vi "HFRR ADV v13.vi"() -> ()   [LabVIEW 2025] (continued)
              }
              frame True {
                n1529 = Delete From Array(array=w2011, length=w2010, index=0) -> (array with subset deleted=w2012:dbl[])  [unwired: 1 out]
                "Numeric" <- w2010
              }
            }
            "FF1" <- w1997
            "PID Ref" <- TRUE ("PID Ref")
          }
          frame #2 {
          }
          frame #3 {
            # "CONVERT TO N"
            # "DATA PROCESSING"
            # "115 mV/N"
            n1530 = local read "RH Numeric:"() -> (w2018:dbl)
            n1531 = local read "HUMIDITY:"() -> (w2019:dbl)
            n1532 = local read "temp buf"() -> (w2080:dbl[])
            n1533 = local read "Air temp"() -> (w2078:dbl[])
            n1534 = local read "ecr buf"() -> (w2040:dbl[])
            n1535 = local read "Fric Val"() -> (w2083:dbl[])
            n1536 = case shown="True" "Reset Button" {
              frame False {
              }
              frame True {
                n1537 = local write "Reset Button"(FALSE) -> ()
                n1538 = local write "Captured Values"(dbl[][] [] ("Captured Values")) -> ()
                n1539 = local write "Best Fit"(dbl[] [] ("Best Fit")) -> ()
              }
            }
            n1540 = local read "TEMPERATURE :"() -> (w2061:dbl)
            n1541 = call-poly <vilib>:"Mean.vi"("X"=w2040) -> ("mean"=w2037:dbl)  [unwired: 1 out]
            n1542 = call-poly <vilib>:"Mean.vi"("X"=w2078) -> ("mean"=w2047:dbl)  [unwired: 1 out]
            "Raw air temp" <- w2047
            n1543 = call-poly <vilib>:"Mean.vi"("X"=w2080) -> ("mean"=w2049:dbl)  [unwired: 1 out]
            "Raw specimen temp" <- w2049
            n1544 = local read "TEMP INTERCEPT:"() -> (w2054:dbl)
            n1545 = Multiply(x=w2018, y=w2019) -> (x*y=→"Humidity ( %RH )" →"Hum" →"Hum 2":dbl)
            n1546 = Multiply(x=w2083, y=1.0) -> (x*y=w2084:dbl[])
            n1547 = local read "FRIC. FORCE :"() -> (w2077:dbl)
            n1548 = Multiply(x=w2049, y=w2061) -> (x*y=w2043:dbl)
            n1549 = local read "AIR TEMPERATURE :"() -> (w2062:dbl)
            n1550 = local read "RUN"() -> (w2074:bool)
            n1551 = Add(x=w2047, y="Offset Air Temp") -> (x+y=w2042:dbl)
            n1552 = local read "AIR TEMP INTERCEPT:"() -> (w2058:dbl)
            n1553 = case shown="\"0\", Default" "Calibrating" {
              tunnel: w2049 -> [w2103 _]
              tunnel: [w2103 w2104] -> w2048
              tunnel: w2047 -> [_ w2104]
              frame "0", Default {
              }
              frame "1" {
              }
            }
            n1554 = Multiply(x=w2037, y="ECR_Gain") -> (x*y=w2036:dbl)
            n1555 = Add(x=w2043, y=w2054) -> (x+y=w2059:dbl)
            n1556 = Multiply(x=w2077, y=79.77669138) -> (x*y=w2075:dbl)
            n1557 = Select(t=0.01 ("FF fil1"), s=w2074, f=0.1 ("FF fil1")) -> (s? t:f=w2070:dbl)
            n1558 = local read "ecr"() -> (w2031:dbl)
            n1559 = Multiply(x=w2042, y=w2062) -> (x*y=w2044:dbl)
            n1560 = Multiply(x=w2084, y=w2075) -> (x*y=w2081:dbl[])
            n1561 = Multiply(x=w2036, y=0.2) -> (x*y=w2029:dbl)
            n1562 = Multiply(x=0.8, y=w2031) -> (x*y=w2030:dbl)
            n1563 = call <vilib>:"Mean PtByPt.vi"("x"=w2059, "sample length"=10) -> ("mean"=w2020:dbl)  [unwired: 2 in, 1 out]
            "TEMP 2" <- w2020
            "TEMP 3" <- w2020
            n1564 = local read "AIR TEMP"() -> (w2067:dbl)
            n1565 = Add(x=w2044, y=w2058) -> (x+y=w2060:dbl)
            n1566 = call-poly <vilib>:"Mean.vi"("X"=w2081) -> ("mean"=w2082:dbl)  [unwired: 1 out]
            n1567 = Add(x=w2029, y=w2030) -> (x+y=w2028:dbl)
            n1568 = Subtract(x=1.0 ("y"), y=w2070) -> (x-y=w2068:dbl)
            n1569 = local write "TEMP"(w2020) -> ()
            n1570 = Multiply(x=w2068, y=w2067) -> (x*y=w2066:dbl)
            n1571 = Multiply(x=w2060, y=w2070) -> (x*y=w2071:dbl)
            n1572 = Not A Number/Path/Refnum?(number/path/refnum=w2028) -> (NaN/Path/Refnum?=w2038:bool)
            n1573 = Subtract(x=w2081, y=w2082) -> (x-y=w2053:dbl[])
            n1574 = local read "FRICVALZ"() -> (w2091:dbl)
            n1575 = case shown="True" "Camera Button" {
              tunnel: w2048 -> [_ w2110]
              tunnel: "Standard Temp. ( °c )" -> [_ w2109]
              frame False {
              }
              frame True {
                n1576 = Build Array(w2109, w2110) -> (w2108:dbl[])
                n1577 = local write "Camera Button"(FALSE ("Boolean 4")) -> ()
                n1578 = local read "Captured Values"() -> (w2107:dbl[][])
                n1579 = Build Array (concatenate)(w2107, w2108) -> (w2105:dbl[][])
                n1580 = local write "Captured Values"(w2105) -> ()
              }
            }
            n1581 = Compound Arithmetic op=OR("FRICVALZ 4", "FRICVALZ 3", "FRICVALZ 2") -> (w2022:bool)
            n1582 = Add(x=w2071, y=w2066) -> (x+y=w2064:dbl)
            n1583 = Absolute Value(x=w2053) -> (abs(x)=w2086:dbl[])
            n1584 = call-poly <vilib>:"RMS.vi"("X"=w2053) -> ("rms value"=w2052:dbl)  [unwired: 1 out]
            n1585 = Select(t=0.0, s=w2038, f=w2028) -> (s? t:f=w2035:dbl)
            n1586 = call-poly <vilib>:"Mean.vi"("X"=w2086) -> ()  [unwired: 2 out]
            n1587 = local read "FF 2"() -> (w2093:dbl)
            n1588 = case shown="True" w2022 {
              tunnel: w2052 -> [_ w2115]
              frame False {
              }
              frame True {
                w2114 = FALSE ("FRICVALZ")
                n1589 = local write "FRICVALZ 3"(w2114) -> ()
                n1590 = local write "FRICVALZ 2"(w2114) -> ()
                n1591 = local write "FRICVALZ 4"(w2114) -> ()
                "FRICVALZ" <- w2115
              }
            }
            n1592 = Subtract(x=w2052, y=w2091) -> (x-y=w2085:dbl)
            n1593 = Not A Number/Path/Refnum?(number/path/refnum=w2064) -> (NaN/Path/Refnum?=w2065:bool)
            n1594 = In Range and Coerce(upper limit=100.0, x=w2035, lower limit=0.0) -> ()  [unwired: 2 out]
            n1595 = Select(t=0.0, s=w2065, f=w2064) -> (s? t:f=w2025:dbl)
            "AIR TEMP" <- w2025
            n1596 = Multiply(x=w2085, y=0.1 ("FF fil1")) -> (x*y=w2097:dbl)
            n1597 = Multiply(x=0.9 ("FF fil2"), y=w2093) -> (x*y=w2096:dbl)
            n1598 = disable-structure shown="Disabled" {
              frame Disabled {
                n1599 = local read "NORMAL LOAD"() -> ()  [unwired: 1 out]
              }
              frame Enabled {
              }
            }
            n1600 = call "Elapsed Time11"("Time Target (s)"=1.0) -> ("Time has Elapsed"=w2027:bool)  [unwired: 11 in, 7 out]
            n1601 = Add(x=w2097, y=w2096) -> (x+y=w2015:dbl)
            "FF 2" <- w2015
            "FF 4" <- w2015
            n1602 = case shown="True" w2027 {
              tunnel: w2025 -> [_ w2099]
              frame False {
              }
              frame True {
                "AirT" <- w2099
              }
            }
            n1603 = local read "TEMP"() -> (w2090:dbl)
            n1604 = local write "FF 3"(w2015) -> ()
            n1605 = Not A Number/Path/Refnum?(number/path/refnum=w2015) -> (NaN/Path/Refnum?=w2088:bool)
            n1606 = Divide(x=w2015, y=1.96) -> (x/y=w2055:dbl)
            n1607 = Not A Number/Path/Refnum?(number/path/refnum=w2090) -> (NaN/Path/Refnum?=w2089:bool)
            n1608 = Compound Arithmetic op=OR(w2089, w2088) -> (w2087:bool)
            n1609 = Not A Number/Path/Refnum?(number/path/refnum=w2055) -> (NaN/Path/Refnum?=w2056:bool)
            n1610 = case shown="True" w2087 {
              frame False {
              }
              frame True {
                n1611 = local write "TEMP"(0.0 ("TEMP")) -> ()
                n1612 = local write "FF 2"(0.0 ("FF 2")) -> ()
                n1613 = local write "reinit"(TRUE ("reinit")) -> ()
              }
            }
            n1614 = Select(t=0.0, s=w2056, f=w2055) -> (s? t:f=w2016:dbl)
            "COF 2" <- w2016
            n1615 = local write "COF 3"(w2016) -> ()
          }
          frame #4 {
            n1616 = flat-sequence {
              frame #0 {
                n1617 = Wait (ms)(milliseconds to wait=u32 100) -> ()  [unwired: 1 out]
              }
              frame #1 {
                n1618 = local write "Lift"(FALSE ("Lift")) -> ()
              }
            }
            n1619 = case shown="True" "Calculate Button" {
              frame False {
              }
              frame True {
                n1620 = local write "Calculate Button"(FALSE ("Boolean 6")) -> ()
                n1621 = local read "Captured Values"() -> (w2126:dbl[][])
                n1622 = Index Array(array=w2126, index (col) #1=0 ("disabled index (col)"), index (col) #2=1 ("index (col)")) -> (element #1=w2124:dbl[], element #2=w2122:dbl[])  [unwired: 2 in]
                n1623 = call <vilib>:"Linear Fit.vi"("Y"=w2124, "X"=w2122) -> ("Best Linear Fit"=→"Best Fit":dbl[], "slope"=w2118:dbl, "intercept"=w2117:dbl)  [unwired: 9 in, 2 out]
                "Slope" <- w2118
                "Intercept" <- w2117
                n1624 = local read "Calibrating"() -> (w2119:string)
                n1625 = case shown="\"1\"" w2119 {
                  tunnel: w2118 -> [w2128 w2130]
                  tunnel: w2117 -> [w2127 w2129]
                  frame "0", Default {
                    n1626 = local write "TEMPERATURE :"(w2128) -> ()
                    n1627 = local write "TEMP INTERCEPT:"(w2127) -> ()
                  }
                  frame "1" {
                    n1628 = local write "AIR TEMPERATURE :"(w2130) -> ()
                    n1629 = local write "AIR TEMP INTERCEPT:"(w2129) -> ()
                  }
                }
              }
            }
          }
        }
      }
    }
    n1630 = Wait (ms)(milliseconds to wait=u32 50) -> ()  [unwired: 1 out]
    n1631 = local read "Quit"() -> (w1920:bool)
    "Rate" <- 2500.0 ("No of Samples")
    "Humid Last buf" <- dbl[] [0.0, 0.0, 0.0, 0.0] ("Humid Last buf")
  }
  n1632 = while {
    tunnel: w60 -> [_]
    tunnel: [w2160] -> _
    tunnel: [w2135] -> w57
    i -> [w2160]
    stop <- w2135 stop-if-true
    # "C:\\LAB-IQ-NXT\\Scar View.exe"
    n1633 = local read "OK Button 16"() -> (w2149:bool)
    n1634 = local read "Re-Initialise"() -> (w2145:bool)
    n1635 = local read "Main Tab"() -> (w2141:T2)
    n1636 = local read "service 3"() -> (w2142:bool)
    n1637 = local read "OPEN 6"() -> (w2144:bool)
    n1638 = local read "EDIT 2"() -> (w2147:bool)
    n1639 = flat-sequence {
      frame #0 {
        n1640 = local read "SAVE 2"() -> (w2763:bool)
        n1641 = stacked-sequence {
          frame #0 {
            n1642 = local read "EDIT"() -> (w2817:bool)
            n1643 = case shown="True" w2817 {
              tunnel: [u8 2 ("Disabled") u8 0 ("Disabled")] -> _
              frame False {
                w2819 = FALSE
                n1644 = local write "Password"("") -> ()
                n1645 = property on="SrvM CP" class="Bool (strict)"("Visible"=w2819) -> ()  [unwired: 2 in, 2 out]
                n1646 = property on="message" class="Str"("Visible"=w2819) -> ()  [unwired: 2 in, 2 out]
                n1647 = local write "x = y?"(w2819) -> ()
                n1648 = property on="Password" class="Str"("Visible"=w2819) -> ()  [unwired: 2 in, 2 out]
                n1649 = property on="ENTER THE NEW PASSWORD" class="Str"("Visible"=w2819) -> ()  [unwired: 2 in, 2 out]
                n1650 = property on="ENTER CURRENT PASSWORD" class="Str"("Visible"=w2819) -> ()  [unwired: 2 in, 2 out]
                n1651 = local write "SrvM CP"(w2819) -> ()
              }
              frame True {
                w2822 = TRUE
                n1652 = property on="SrvM CP" class="Bool (strict)"("Visible"=w2822) -> ()  [unwired: 2 in, 2 out]
                n1653 = property on="Password" class="Str"("Visible"=w2822) -> ()  [unwired: 2 in, 2 out]
              }
            }
            "dipl pwd" <- "@143$\n" ("dipl pwd")
          }
          frame #1 {
            # "Gain password"
            n1654 = String To Byte Array(string="ENTER CURRENT PASSWORD") -> (unsigned byte array=w2827:u8[])
            n1655 = Search 1D Array(1D array=w2827, element=u8 10) -> (index of element=w2830:i32)  [unwired: 1 in]
            n1656 = Index Array(array=w2827, index=w2830) -> (element=w2826:u8)
            n1657 = Equal?(x=w2826, y=10) -> (x = y?=w2824:bool)
            n1658 = case shown="True" w2824 {
              frame False {
                n1659 = property on="ENTER THE NEW PASSWORD" class="Str"("Visible"=FALSE) -> ()  [unwired: 2 in, 2 out]
              }
              frame True {
                # "password"
                # "change password logic"
                n1660 = local read "ENTER CURRENT PASSWORD"() -> (w2843:string)
                n1661 = local read "dipl pwd"() -> (w2837:string)
                n1662 = String To Byte Array(string=w2843) -> (unsigned byte array=w2845:u8[])
                n1663 = String To Byte Array(string=w2837) -> (unsigned byte array=w2838:u8[])
                n1664 = Array Size(array=w2845) -> (size(s)=w2842:i32)
                n1665 = Array Size(array=w2838) -> (size(s)=w2840:i32)
                n1666 = for {
                  N: w2842 -> [_]
                  tunnel: w2845 -> [w2869]
                  tunnel: [w2867] -> w2846 mode=indexing
                  tunnel: w2842 -> [w2861]
                  i -> [w2862]
                  n1667 = Decrement(x=w2861) -> (x-1=w2859:i32)
                  n1668 = Equal?(x=w2862, y=w2859) -> (x = y?=w2860:bool)
                  n1669 = Index Array(array=w2869, index=w2862) -> (element=w2863:u8)
                  n1670 = Number To Decimal String(number=w2863) -> (decimal integer string=w2868:string)  [unwired: 1 in]
                  n1671 = Select(t="", s=w2860, f="\r") -> (s? t:f=w2865:string)
                  n1672 = Concatenate Strings(w2868, w2865) -> (w2867:string)
                }
                n1673 = for {
                  N: w2840 -> [_]
                  tunnel: w2838 -> [w2857]
                  tunnel: [w2855] -> w2839 mode=indexing
                  tunnel: w2840 -> [w2852]
                  i -> [w2853]
                  n1674 = Decrement(x=w2852) -> (x-1=w2851:i32)
                  n1675 = Equal?(x=w2853, y=w2851) -> (x = y?=w2850:bool)
                  n1676 = Index Array(array=w2857, index=w2853) -> (element=w2856:u8)
                  n1677 = Number To Decimal String(number=w2856) -> (decimal integer string=w2854:string)  [unwired: 1 in]
                  n1678 = Select(t="", s=w2850, f="\r") -> (s? t:f=w2847:string)
                  n1679 = Concatenate Strings(w2854, w2847) -> (w2855:string)
                }
                n1680 = local read "string"() -> (w2844:string)
                n1681 = Concatenate Strings(w2839) -> (w2833:string)
                n1682 = Concatenate Strings(w2844) -> (w2841:string)
                n1683 = Concatenate Strings(w2846) -> (w2834:string)
                n1684 = Equal?(x=w2834, y=w2841) -> (x = y?=w2836:bool)
                n1685 = Equal?(x=w2834, y=w2833) -> (x = y?=w2832:bool)
                n1686 = Or(x=w2836, y=w2832) -> (x .or. y?=w2835:bool)
                n1687 = case shown="True" w2835 {
                  frame False {
                  }
                  frame True {
                    n1688 = property on="ENTER THE NEW PASSWORD" class="Str"("Visible"=TRUE) -> ()  [unwired: 2 in, 2 out]
                  }
                }
              }
            }
          }
          frame #2 {
            n1689 = String To Byte Array(string="ENTER THE NEW PASSWORD") -> (unsigned byte array=w2872:u8[])
            n1690 = Search 1D Array(1D array=w2872, element=u8 10) -> (index of element=w2876:i32)  [unwired: 1 in]
            n1691 = Index Array(array=w2872, index=w2876) -> (element=w2874:u8)
            n1692 = Equal?(x=w2874, y=10) -> (x = y?=w2871:bool)
            n1693 = case shown="False" w2871 {
              frame False {
              }
              frame True {
                n1694 = local write "EDIT"(FALSE) -> ()
                n1695 = local write "SrvM CP"(FALSE) -> ()
                n1696 = local read "ENTER THE NEW PASSWORD"() -> (w2879:string)
                n1697 = String To Byte Array(string=w2879) -> (unsigned byte array=w2884:u8[])
                n1698 = Array Size(array=w2884) -> (size(s)=w2881:i32)
                n1699 = for {
                  N: w2881 -> [_]
                  tunnel: w2884 -> [w2897]
                  tunnel: [w2894] -> w2886 mode=indexing
                  tunnel: w2881 -> [w2889]
                  i -> [w2887]
                  n1700 = Decrement(x=w2889) -> (x-1=w2890:i32)
                  n1701 = Equal?(x=w2887, y=w2890) -> (x = y?=w2891:bool)
                  n1702 = Index Array(array=w2897, index=w2887) -> (element=w2896:u8)
                  n1703 = Number To Decimal String(number=w2896) -> (decimal integer string=w2895:string)  [unwired: 1 in]
                  n1704 = Select(t="", s=w2891, f="\r") -> (s? t:f=w2888:string)
                  n1705 = Concatenate Strings(w2895, w2888) -> (w2894:string)
                }
                n1706 = local read "file path"() -> (w2878:path)
                n1707 = Concatenate Strings(w2886) -> (w2880:string)
                n1708 = Delete(path (use dialog)=w2878) -> (deleted path=w2882:path)  [unwired: 4 in, 2 out]
                n1709 = call <vilib>:"Write Characters To File.vi"("append to file? (new file:F)"=FALSE, "character string"=w2880, "file path (dialog if empty)"=w2882) -> ()  [unwired: 2 in, 1 out]
              }
            }
          }
          frame #3 {
            n1710 = case shown="True" "SrvM CP" {
              frame False {
                w2900 = ""
                n1711 = local write "ENTER CURRENT PASSWORD"(w2900) -> ()
                n1712 = local write "ENTER THE NEW PASSWORD"(w2900) -> ()
                n1713 = property on="ENTER CURRENT PASSWORD" class="Str"("Visible"=FALSE) -> ()  [unwired: 2 in, 2 out]
              }
              frame True {
                n1714 = property on="ENTER THE NEW PASSWORD" class="Str"() -> ("Visible"=w2901:bool)  [unwired: 2 in, 2 out]
                n1715 = Not(x=w2901) -> (.not. x?=w2902:bool)
                n1716 = property on="ENTER CURRENT PASSWORD" class="Str"("Visible"=w2902) -> ()  [unwired: 2 in, 2 out]
              }
            }
          }
          frame #4 {
            n1717 = String To Byte Array(string="Password") -> (unsigned byte array=w2909:u8[])
            n1718 = Search 1D Array(1D array=w2909, element=u8 10) -> (index of element=w2907:i32)  [unwired: 1 in]
            n1719 = Index Array(array=w2909, index=w2907) -> (element=w2908:u8)
            n1720 = Equal?(x=w2908, y=10) -> (x = y?=w2904:bool)
            n1721 = case shown="True" w2904 {
              frame False {
              }
              frame True {
                # "password"
                # "password"
                n1722 = local read "Password"() -> (w2922:string)
                n1723 = String To Byte Array(string=w2922) -> (unsigned byte array=w2925:u8[])
                n1724 = String To Byte Array(string="@143$\n") -> (unsigned byte array=w2911:u8[])
                n1725 = Array Size(array=w2925) -> (size(s)=w2920:i32)
                n1726 = Array Size(array=w2911) -> (size(s)=w2916:i32)
                n1727 = for {
                  N: w2920 -> [_]
                  tunnel: w2925 -> [w2959]
                  tunnel: [w2957] -> w2926 mode=indexing
                  tunnel: w2920 -> [w2954]
                  i -> [w2955]
                  n1728 = Decrement(x=w2954) -> (x-1=w2953:i32)
                  n1729 = Index Array(array=w2959, index=w2955) -> (element=w2958:u8)
                  n1730 = Equal?(x=w2955, y=w2953) -> (x = y?=w2952:bool)
                  n1731 = Number To Decimal String(number=w2958) -> (decimal integer string=w2956:string)  [unwired: 1 in]
                  n1732 = Select(t="", s=w2952, f="\r") -> (s? t:f=w2949:string)
                  n1733 = Concatenate Strings(w2956, w2949) -> (w2957:string)
                }
                n1734 = for {
                  N: w2916 -> [_]
                  tunnel: w2911 -> [w2970]
                  tunnel: [w2968] -> w2914 mode=indexing
                  tunnel: w2916 -> [w2965]
                  i -> [w2966]
                  n1735 = Decrement(x=w2965) -> (x-1=w2964:i32)
                  n1736 = Index Array(array=w2970, index=w2966) -> (element=w2969:u8)
                  n1737 = Equal?(x=w2966, y=w2964) -> (x = y?=w2963:bool)
                  n1738 = Number To Decimal String(number=w2969) -> (decimal integer string=w2967:string)  [unwired: 1 in]
                  n1739 = Select(t="", s=w2963, f="\r") -> (s? t:f=w2960:string)
                  n1740 = Concatenate Strings(w2967, w2960) -> (w2968:string)
                }
                n1741 = local read "file path"() -> (w2910:path)
                n1742 = call <vilib>:"Read Characters From File.vi"("file path (dialog if empty)"=w2910) -> ("character string"=w2924:string)  [unwired: 5 in, 3 out]
                "string" <- w2924
                n1743 = flat-sequence {
                  tunnel: [w2927] -> w2921
                  frame #0 {
                    w2927 = ""
                    n1744 = local write "Password"(w2927) -> ()
                  }
                }
                n1745 = Concatenate Strings(w2914) -> (w2915:string)
                n1746 = Concatenate Strings(w2924) -> (w2923:string)
                n1747 = Concatenate Strings(w2926) -> (w2918:string)
                n1748 = Equal?(x=w2918, y=w2923) -> (x = y?=w2913:bool)
                n1749 = Equal?(x=w2918, y=w2915) -> (x = y?=w2919:bool)
                n1750 = Or(x=w2913, y=w2919) -> (x .or. y?=w2912:bool)
                "x = y?" <- w2912
                n1751 = case shown="True" w2912 {
                  selector: w2912 -> [w2929 _]
                  tunnel: w2921 -> [_ _]
                  frame False {
                    n1752 = And(x=w2929, y=TRUE ("Visible")) -> (x .and. y?=w2930:bool)
                    n1753 = property on="message" class="Str"("Visible"=w2930) -> ()  [unwired: 2 in, 2 out]
                  }
                  frame True {
                    n1754 = control-ref of="This VI"() -> (w2941:refnum<vi>)
                    n1755 = property class="VI"(reference=w2941) -> (reference out=w2932:refnum<vi>, error out=w2936:errorcluster, "Panel"=w2940:refnum<vi>)  [unwired: 1 in]
                    n1756 = property on="message" class="Str"("Visible"=FALSE) -> ()  [unwired: 2 in, 2 out]
                    n1757 = property class="Pnl"(reference=w2940, error in=w2936) -> (reference out=w2934:refnum<vi>, error out=w2937:errorcluster, "Panes[]"=w2939:refnum<vi>[])
                    n1758 = for {
                      tunnel: w2939 -> [w2948] mode=indexing
                      tunnel: T18."Always On" ("Horizontal Scrollbar Visibility") -> [w2947]
                      tunnel: w2937 -> [w2944]
                      tunnel: [w2943] -> w2935
                      n1759 = property class="Pane"(reference=w2948, error in=w2944, "HorizScrollbarVisibility"=w2947) -> (reference out=w2945:refnum<vi>, error out=w2946:errorcluster)
                      n1760 = Close Reference(reference=w2945, error in (no error)=w2946) -> (error out=w2943:errorcluster)
                    }
                    n1761 = Close Reference(reference=w2934, error in (no error)=w2935) -> (error out=w2933:errorcluster)
                    n1762 = Close Reference(reference=w2932, error in (no error)=w2933) -> (error out=→"error out 6":errorcluster)
                  }
                }
              }
            }
          }
        }
        n1763 = local read "x = y?"() -> (w2769:bool)
        n1764 = local read "HUMIDITY: 2"() -> (w2771:dbl)
        n1765 = local read "HUMIDITY:"() -> (w2770:dbl)
        n1766 = property on="Port 2 Error" class="Clust (strict)"("Visible"="EDIT") -> ()  [unwired: 2 in, 2 out]
        n1767 = property on="Port 1 Error" class="Clust (strict)"("Visible"="EDIT") -> ()  [unwired: 2 in, 2 out]
        n1768 = case shown="True" "SrvM CP 2" {
          frame False {
          }
          frame True {
            n1769 = local write "SrvM CP 2"(FALSE ("SrvM CP 2")) -> ()
            n1770 = local read "HUMIDITY: 2"() -> (w2810:dbl)
            n1771 = local read "TEMP INTERCEPT: 2"() -> (w2809:dbl)
            n1772 = local read "DISPLACEMENT : 4"() -> (w2813:dbl)
            n1773 = local read "TEMPERATURE : 2"() -> (w2812:dbl)
            n1774 = local read "STROKE GAIN : 2"() -> (w2814:dbl)
            n1775 = local read "FRIC. FORCE : 2"() -> (w2815:dbl)
            n1776 = local read "AIR TEMP INTERCEPT: 2"() -> (w2808:dbl)
            n1777 = local read "AIR TEMPERATURE : 2"() -> (w2811:dbl)
            n1778 = local write "HUMIDITY:"(w2810) -> ()
            n1779 = local write "AIR TEMP INTERCEPT:"(w2809) -> ()
            n1780 = local write "TEMPERATURE :"(w2812) -> ()
            n1781 = local write "FRIC. FORCE :"(w2815) -> ()
            n1782 = local write "STROKE GAIN :"(w2814) -> ()
            n1783 = local write "DISPLACEMENT :"(w2813) -> ()
            n1784 = local write "AIR TEMPERATURE :"(w2811) -> ()
            n1785 = local write "TEMP INTERCEPT:"(w2808) -> ()
          }
        }
        n1786 = Or(x="SAVE", y=w2763) -> (x .or. y?=w2764:bool)
        n1787 = And(x="EDIT", y=w2769) -> (x .and. y?=w2767:bool)
        n1788 = local read "DISPLACEMENT : 4"() -> (w2780:dbl)
        n1789 = local read "TEMPERATURE : 2"() -> (w2778:dbl)
        n1790 = local read "STROKE GAIN : 2"() -> (w2784:dbl)
        n1791 = local read "DISPLACEMENT :"() -> (w2779:dbl)
        n1792 = local read "FRIC. FORCE : 2"() -> (w2787:dbl)
        n1793 = local read "TEMPERATURE :"() -> (w2776:dbl)
        n1794 = local read "STROKE GAIN :"() -> (w2783:dbl)
        n1795 = local read "FRIC. FORCE :"() -> (w2786:dbl)
        n1796 = case shown="True" w2767 {
          tunnel: [u8 2 ("Disabled") u8 0 ("Disabled")] -> w2766
          tunnel: [w3157 TRUE ("Visible")] -> w2765
          frame False {
            w3157 = FALSE ("Visible")
            n1797 = local write "EDIT 2"(w3157) -> ()
          }
          frame True {
          }
        }
        n1798 = case shown="True" w2764 {
          frame False {
          }
          frame True {
            n1799 = stacked-sequence {
              seq-local: [w2987 _ _] -> [_ w3151 _]
              frame #0 {
                (unwired) i16 5 ("precision (6)")
                # "[CH1]    - FF\n[CH2]   - TEMPERATURE\n[CH3]    - Humidity\n[CH4]    - AIR TEMP\n[CH5]\\- Visa Uno\n[CH6] \\- Visa Due\n[CH7]  \\- file path\n[CH8]   - Displacement Gain\n[CHA]   - Stroke Gain\n[CHB]   - Stroke PID Gain\n[CHC]   -Language Selection\n[CHD]   -Power +\n[CHE]   -Power_\n[CHF]   -Heater\n[CHG]   -Humidity Wet\n[CHH]   -Humidity Dry\n[CHI]   -Integral Time"
                n1800 = local read "Stroke PID Gains"() -> (w3038:T9)
                n1801 = Unbundle By Name(w3038) -> ("Proportional Gain (Kc)"=w3037:dbl, "Integral Time (Ti, min)"=w2979:dbl)
                n1802 = Number To Fractional String(number=w2979, width (-)=i16 10 ("precision (6)"), precision (6)=i16 5) -> (F-format string=w2983:string)  [unwired: 1 in]
                n1803 = local read "Language Selection"() -> (w3035:enum16{"English", "Russian"})
                n1804 = local read "CH-HUMIDITY WET"() -> (w2993:u16)
                n1805 = local read "CH-HUMIDITY DRY"() -> (w2990:u16)
                n1806 = local read "STROKE GAIN :"() -> (w2971:dbl)
                n1807 = local read "CH-POWER +"() -> (w3002:u16)
                n1808 = local read "CH-POWER -"() -> (w2999:u16)
                n1809 = local read "CH-HEATER"() -> (w2996:u16)
                n1810 = local read "AIR TEMPERATURE :"() -> (w2974:dbl)
                n1811 = Concatenate Strings("[CHI]" ("string"), w2983, "-Integral Time " ("string"), "\r") -> (w2980:string)
                n1812 = local read "DISPLACEMENT :"() -> (w2972:dbl)
                n1813 = local read "TEMPERATURE :"() -> (w2975:dbl)
                n1814 = local read "FRIC. FORCE :"() -> (w2976:dbl)
                n1815 = local read "HUMIDITY:"() -> (w2973:dbl)
                n1816 = Path To String(path="File Path") -> (string=w3060:string)
                n1817 = Number To Fractional String(number=w2971, width (-)=i16 10 ("precision (6)"), precision (6)=i16 5) -> (F-format string=w3051:string)  [unwired: 1 in]
                n1818 = Number To Fractional String(number=w3037, width (-)=i16 10 ("precision (6)"), precision (6)=i16 5) -> (F-format string=w3039:string)  [unwired: 1 in]
                n1819 = Number To Fractional String(number=w3035, width (-)=i16 10 ("precision (6)"), precision (6)=i16 5) -> (F-format string=w3031:string)  [unwired: 1 in]
                n1820 = Number To Fractional String(number=w3002, width (-)=i16 10 ("precision (6)"), precision (6)=i16 5) -> (F-format string=w3025:string)  [unwired: 1 in]
                n1821 = Number To Fractional String(number=w2999, width (-)=i16 10 ("precision (6)"), precision (6)=i16 5) -> (F-format string=w3022:string)  [unwired: 1 in]
                n1822 = Number To Fractional String(number=w2996, width (-)=i16 10 ("precision (6)"), precision (6)=i16 5) -> (F-format string=w3017:string)  [unwired: 1 in]
                n1823 = Number To Fractional String(number=w2993, width (-)=i16 10 ("precision (6)"), precision (6)=i16 5) -> (F-format string=w3014:string)  [unwired: 1 in]
                n1824 = Number To Fractional String(number=w2990, width (-)=i16 10 ("precision (6)"), precision (6)=i16 5) -> (F-format string=w3009:string)  [unwired: 1 in]
                n1825 = local read "Com Port 1"() -> (w2978:refnum<visa-resource-name>)
                n1826 = local read "Com Port 2"() -> (w2977:refnum<visa-resource-name>)
                n1827 = Concatenate Strings(w3060, "\\" ("string")) -> (w3059:string)
                n1828 = Number To Fractional String(number=w2976, width (-)=i16 10 ("precision (6)"), precision (6)=i16 5) -> (F-format string=w3092:string)  [unwired: 1 in]
                n1829 = Number To Fractional String(number=w2975, width (-)=i16 10 ("precision (6)"), precision (6)=i16 5) -> (F-format string=w3091:string)  [unwired: 1 in]
                n1830 = Number To Fractional String(number=w2973, width (-)=i16 10 ("precision (6)"), precision (6)=i16 5) -> (F-format string=w3085:string)  [unwired: 1 in]
                n1831 = Number To Fractional String(number=w2974, width (-)=i16 10 ("precision (6)"), precision (6)=i16 5) -> (F-format string=w3079:string)  [unwired: 1 in]
                n1832 = Number To Fractional String(number=w2972, width (-)=i16 10 ("precision (6)"), precision (6)=i16 5) -> (F-format string=w3052:string)  [unwired: 1 in]
                n1833 = Concatenate Strings("[CHA]" ("string"), w3051, "- Stroke Gain" ("string"), "\r") -> (w3045:string)
                n1834 = Concatenate Strings("[CHB]" ("string"), w3039, "- Stroke PID Gain" ("string"), "\r") -> (w3036:string)
                n1835 = Concatenate Strings("[CHC]" ("string"), w3031, "-Language Selection" ("string"), "\r") -> (w3028:string)
                n1836 = Concatenate Strings("[CHD]" ("string"), w3025, "-Power +" ("string"), "\r") -> (w3007:string)
                n1837 = Concatenate Strings("[CHG]" ("string"), w3014, "-Humidity Wet" ("string"), "\r") -> (w3004:string)
                n1838 = Concatenate Strings("[CHH]" ("string"), w3009, "-Humidity Dry" ("string"), "\r") -> (w3003:string)
                n1839 = Concatenate Strings("[CH1]" ("string"), w3092, " - FF" ("string"), "\r") -> (w3090:string)
                n1840 = Concatenate Strings("[CH2]" ("string"), w3091, " - TEMPERATURE" ("string"), "\r") -> (w3089:string)
                n1841 = Concatenate Strings("[CH3]" ("string"), w3085, " - Humidity" ("string"), "\r") -> (w3082:string)
                n1842 = Concatenate Strings("[CH4]" ("string"), w3079, " - AIR TEMP" ("string"), "\r") -> (w3075:string)
                n1843 = Concatenate Strings("[CH5]" ("string"), w2978, "- Visa Uno" ("string"), "\r") -> (w3068:string)
                n1844 = Concatenate Strings("[CH6]" ("string"), w2977, "- Visa Due" ("string"), "\r") -> (w3063:string)
                n1845 = Concatenate Strings("[CH7]" ("string"), w3059, "- file path" ("string"), "\r") -> (w3062:string)
                n1846 = Concatenate Strings("[CH8]" ("string"), w3052, "- Displacement Gain" ("string"), "\r") -> (w3055:string)
                n1847 = Concatenate Strings("[CHE]" ("string"), w3022, "-Power_" ("string"), "\r") -> (w3006:string)
                n1848 = Concatenate Strings("[CHF]" ("string"), w3017, "-Heater" ("string"), "\r") -> (w3005:string)
                n1849 = Concatenate Strings(w3090, w3089, w3082, w3075, w3068, w3063, w3062, w3055, w3045, w3036, w3028, w3007, w3006, w3005, w3004, w3003, w2980) -> (w2987:string)
                "gain" <- w2987
              }
              frame #1 {
                n1850 = local read "Camera Port :"() -> (w3104:string)
                n1851 = local read "TEMP INTERCEPT:"() -> (w3113:dbl)
                n1852 = local read "AIR TEMP INTERCEPT:"() -> (w3114:dbl)
                n1853 = local read "C3 :"() -> (w3112:refnum<visa-resource-name>)
                n1854 = local read "LvdtOff"() -> (w3116:dbl)
                n1855 = Number To Fractional String(number=w3113, width (-)=i16 10 ("precision (6)"), precision (6)=i16 5) -> (F-format string=w3139:string)  [unwired: 1 in]
                n1856 = local read "Com Port 3"() -> (w3123:refnum<visa-resource-name>)
                n1857 = Concatenate Strings("[CH8]" ("string"), w3104, "- Visa Camera" ("string"), "\r") -> (w3103:string)
                n1858 = Concatenate Strings("[CH7]" ("string"), w3112, "- Visa Humidity" ("string"), "\r") -> (w3108:string)
                n1859 = Number To Fractional String(number=w3114, width (-)=i16 10 ("precision (6)"), precision (6)=i16 5) -> (F-format string=w3146:string)  [unwired: 1 in]
                n1860 = Number To Fractional String(number=w3116, width (-)=i16 10 ("precision (6)"), precision (6)=i16 5) -> (F-format string=w3120:string)  [unwired: 1 in]
                n1861 = Concatenate Strings("[CHK]" ("string"), w3139, "-TEMP INTERCEPT" ("string"), "\r") -> (w3135:string)
                n1862 = Concatenate Strings("[SNO]" ("string"), "S.NO", "-" ("string"), "\r") -> (w3131:string)
                n1863 = Concatenate Strings("[CHI]" ("string"), w3120, "-LVDT Position Offset" ("string"), "\r") -> (w3115:string)
                n1864 = Concatenate Strings("[CHJ]" ("string"), w3146, "-AIR TEMP INTERCEPT" ("string"), "\r") -> (w3136:string)
                n1865 = Concatenate Strings("[CHL]" ("string"), w3123, "- Visa humid" ("string"), "\r") -> (w3126:string)
                n1866 = String To Path(string="C:\\LAB-IQ\\calibrate WO 2465.dcf") -> (path=w3124:path)
                n1867 = Concatenate Strings(w3151, w3136, w3135, w3131, w3126, w3115, w3108, w3103) -> (w3150:string)
                n1868 = call <vilib>:"Write Characters To File.vi"("append to file? (new file:F)"=FALSE, "character string"=w3150, "file path (dialog if empty)"=w3124) -> ()  [unwired: 2 in, 1 out]
              }
              frame #2 {
                n1869 = local write "Lan flag"(0.0 ("Lan flag")) -> ()
                n1870 = local write "conststatus"(0.0 ("rpm value : 2")) -> ()
                n1871 = local write "SAVE"(FALSE ("OK Button 14")) -> ()
                n1872 = local write "Re-Initialise"(TRUE ("Re-Initialise")) -> ()
                n1873 = local write "SAVE 2"(FALSE ("SAVE 2")) -> ()
              }
            }
          }
        }
        n1874 = Subtract(x=w2771, y=w2770) -> (x-y=w2772:dbl)
        n1875 = local read "AIR TEMPERATURE : 2"() -> (w2775:dbl)
        n1876 = local read "AIR TEMPERATURE :"() -> (w2774:dbl)
        n1877 = Divide(x=w2772, y=w2770) -> (x/y=w2794:dbl)
        n1878 = Subtract(x=w2787, y=w2786) -> (x-y=w2785:dbl)
        n1879 = Subtract(x=w2778, y=w2776) -> (x-y=w2777:dbl)
        n1880 = Subtract(x=w2784, y=w2783) -> (x-y=w2782:dbl)
        n1881 = Subtract(x=w2780, y=w2779) -> (x-y=w2781:dbl)
        n1882 = Subtract(x=w2775, y=w2774) -> (x-y=w2773:dbl)
        n1883 = Divide(x=w2785, y=w2786) -> (x/y=w2805:dbl)
        n1884 = Divide(x=w2777, y=w2776) -> (x/y=w2798:dbl)
        n1885 = Divide(x=w2782, y=w2783) -> (x/y=w2802:dbl)
        n1886 = Divide(x=w2781, y=w2779) -> (x/y=w2801:dbl)
        n1887 = Multiply(x=w2794, y=100.0) -> (x*y=→"HUMIDITY  Calibration Error":dbl)
        n1888 = Divide(x=w2773, y=w2774) -> (x/y=w2797:dbl)
        n1889 = Multiply(x=w2805, y=100.0) -> (x*y=→"FRIC. FORCE Calibration Error":dbl)
        n1890 = Multiply(x=w2798, y=100.0) -> (x*y=→"TEMPERATURE  Calibration Error":dbl)
        n1891 = Multiply(x=w2802, y=100.0) -> (x*y=→"STROKE Calibration Error":dbl)
        n1892 = Multiply(x=w2801, y=100.0) -> (x*y=→"DISPLACEMENT  Calibration Error":dbl)
        n1893 = property on="EDIT 2" class="Bool (strict)"("Visible"=w2765) -> ()  [unwired: 2 in, 2 out]
        n1894 = property on="SAVE" class="Bool (strict)"("Visible"=w2765) -> ()  [unwired: 2 in, 2 out]
        n1895 = property on="SrvM CP" class="Bool (strict)"("Disabled"=w2766) -> ()  [unwired: 2 in, 2 out]
        n1896 = property on="visa due" class="CmbBox"("Disabled"=w2766) -> ()  [unwired: 2 in, 2 out]
        n1897 = property on="LvdtOff" class="DigNum (strict)"("Disabled"=w2766) -> ()  [unwired: 2 in, 2 out]
        n1898 = property on="File Path" class="Path"("Disabled"=w2766) -> ()  [unwired: 2 in, 2 out]
        n1899 = Multiply(x=w2797, y=100.0) -> (x*y=→"AIR TEMPERATURE  Calibration Error":dbl)
        n1900 = property on="Tab Control" class="TabCtl (strict)"("Visible"=w2765) -> ()  [unwired: 2 in, 2 out]
        n1901 = property on="Language Selection" class="Enum (strict)"("Visible"=w2765) -> ()  [unwired: 2 in, 2 out]
        n1902 = property on="Tab Control 7" class="TabCtl (strict)"("Disabled"=w2766) -> ()  [unwired: 2 in, 2 out]
        n1903 = property on="AIR TEMP INTERCEPT:" class="DigNum (strict)"("Disabled"=w2766) -> ()  [unwired: 2 in, 2 out]
        n1904 = property on="CH-POWER -" class="DigNum (strict)"("Disabled"=w2766) -> ()  [unwired: 2 in, 2 out]
        n1905 = property on="CH-POWER +" class="DigNum (strict)"("Disabled"=w2766) -> ()  [unwired: 2 in, 2 out]
        n1906 = property on="AIR TEMPERATURE :" class="DigNum (strict)"("Disabled"=w2766) -> ()  [unwired: 2 in, 2 out]
        n1907 = property on="STROKE GAIN :" class="DigNum (strict)"("Disabled"=w2766) -> ()  [unwired: 2 in, 2 out]
        n1908 = property on="SPEED OUT:" class="DigNum (strict)"("Disabled"=w2766) -> ()  [unwired: 2 in, 2 out]
        n1909 = property on="CH-HUMIDITY DRY" class="DigNum (strict)"("Disabled"=w2766) -> ()  [unwired: 2 in, 2 out]
        n1910 = property on="HUMIDITY:" class="DigNum (strict)"("Disabled"=w2766) -> ()  [unwired: 2 in, 2 out]
        n1911 = property on="CH-HUMIDITY WET" class="DigNum (strict)"("Disabled"=w2766) -> ()  [unwired: 2 in, 2 out]
        n1912 = property on="Stroke PID Gains" class="Clust (strict)"("Disabled"=w2766) -> ()  [unwired: 2 in, 2 out]
        n1913 = property on="TEMPERATURE :" class="DigNum (strict)"("Disabled"=w2766) -> ()  [unwired: 2 in, 2 out]
        n1914 = property on="DISPLACEMENT :" class="DigNum (strict)"("Disabled"=w2766) -> ()  [unwired: 2 in, 2 out]
        n1915 = property on="CH-HEATER" class="DigNum (strict)"("Disabled"=w2766) -> ()  [unwired: 2 in, 2 out]
        n1916 = property on="TEMP INTERCEPT:" class="DigNum (strict)"("Disabled"=w2766) -> ()  [unwired: 2 in, 2 out]
        n1917 = property on="FRIC. FORCE :" class="DigNum (strict)"("Disabled"=w2766) -> ()  [unwired: 2 in, 2 out]
      }
    }
    n1918 = local read "RUN"() -> (w2159:bool)
    n1919 = local read "RUN"() -> (w2157:bool)
    n1920 = disable-structure shown="Disabled" {
      disable-tunnel: [w2174 _] -> w2139
      disable-tunnel: [w2173 _] -> w2137
      frame Disabled {
        n1921 = local read "Temperature before test"() -> (w2167:dbl)
        n1922 = local read "Temperature after test"() -> (w2180:dbl)
        n1923 = case shown="True" "Save Results" {
          frame False {
          }
          frame True {
            w2196 = "\r"
            n1924 = local write "Save Results"(FALSE ("OK Button 5")) -> ()
            n1925 = local read "Temperature before test"() -> (w2234:dbl)
            n1926 = local read "Temperature after test"() -> (w2236:dbl)
            n1927 = local read "Humidity before test"() -> (w2233:dbl)
            n1928 = local read "Humidity after test"() -> (w2235:dbl)
            n1929 = local read "WS1.4"() -> (w2240:dbl)
            n1930 = local read "AVP"() -> (w2238:dbl)
            n1931 = Number To Fractional String(number=w2240, width (-)=i16 6, precision (6)=i16 1) -> (F-format string=w2200:string)  [unwired: 1 in]
            n1932 = local read "MWSD"() -> (w2237:dbl)
            n1933 = local read "String"() -> (w2229:string)
            n1934 = local read "FILE"() -> (w2232:string)
            n1935 = local read "HCF"() -> (w2239:dbl)
            n1936 = Number To Fractional String(number=w2233, width (-)=i16 6, precision (6)=i16 1) -> (F-format string=w2225:string)  [unwired: 1 in]
            n1937 = Number To Fractional String(number=w2234, width (-)=i16 6, precision (6)=i16 1) -> (F-format string=w2222:string)  [unwired: 1 in]
            n1938 = Number To Fractional String(number=w2235, width (-)=i16 6, precision (6)=i16 1) -> (F-format string=w2218:string)  [unwired: 1 in]
            n1939 = Number To Fractional String(number=w2236, width (-)=i16 6, precision (6)=i16 1) -> (F-format string=w2214:string)  [unwired: 1 in]
            n1940 = Number To Fractional String(number=w2238, width (-)=i16 6, precision (6)=i16 3) -> (F-format string=w2207:string)  [unwired: 1 in]
            n1941 = Concatenate Strings(w2229, w2232) -> (w2251:string)
            n1942 = Number To Fractional String(number=w2237, width (-)=i16 6, precision (6)=i16 1) -> (F-format string=w2211:string)  [unwired: 1 in]
            n1943 = Number To Fractional String(number=w2239, width (-)=i16 6, precision (6)=i16 2) -> (F-format string=w2205:string)  [unwired: 1 in]
            n1944 = Concatenate Strings("(" ("string"), w2200, ")Microns" ("string")) -> (w2199:string)
            n1945 = local read "REMARKS"() -> (w2231:string)
            "REMARKS 2" <- w2231
            n1946 = Concatenate Strings("(" ("string"), w2225, " ) % RH," ("string")) -> (w2226:string)
            n1947 = Concatenate Strings(w2205, ")" ("string")) -> (w2203:string)
            n1948 = Concatenate Strings("(" ("string"), w2222, ")  Deg C ," ("string")) -> (w2221:string)
            n1949 = Concatenate Strings("(" ("string"), w2218, " ) % RH," ("string")) -> (w2217:string)
            n1950 = Concatenate Strings("(" ("string"), w2214, ")  Deg C ," ("string")) -> (w2213:string)
            n1951 = Concatenate Strings("(" ("string"), w2211, ")  Microns," ("string")) -> (w2210:string)
            n1952 = Concatenate Strings("(" ("string"), w2207, ")  kPa," ("string")) -> (w2197:string)
            n1953 = Concatenate Strings(w2251, ".dwm" ("Substring")) -> (w2249:string)
            n1954 = String To Path(string=w2249) -> (path=w2248:path)
            n1955 = Concatenate Strings(w2231, w2196, " Humidity before test= " ("Substring"), w2226, w2196, " Temperature before test = " ("Substring"), w2221, w2196, " Humidity after test= " ("Substring"), w2217, w2196, "Temperature after test = " ("Substring"), w2213, w2196, "MSD = " ("Substring"), w2210, w2196, "  AVP = " ("Substring"), w2197, w2196, "  HCF                     =( " ("Substring"), w2203, w2196, " WS1.4                  = " ("Substring"), w2199, w2196) -> (w2195:string)
            "data" <- w2195
            n1956 = call <vilib>:"Write Characters To File.vi"("append to file? (new file:F)"=FALSE, "character string"=w2195, "file path (dialog if empty)"=w2248) -> ()  [unwired: 2 in, 1 out]
            n1957 = Match Pattern(string=w2195, regular expression="!") -> (after substring=→"export":string)  [unwired: 1 in, 3 out]
          }
        }
        n1958 = Add(x=231.864, y=w2167) -> (x+y=w2164:dbl)
        n1959 = Add(x=231.864, y=w2180) -> (x+y=w2177:dbl)
        n1960 = Divide(x=1705.984, y=w2164) -> (x/y=w2165:dbl)
        n1961 = Divide(x=1705.984, y=w2177) -> (x/y=w2178:dbl)
        n1962 = local read "Humidity before test"() -> (w2169:dbl)
        n1963 = local read "Humidity after test"() -> (w2182:dbl)
        n1964 = Subtract(x=8.017352 ("y"), y=w2165) -> (x-y=w2191:dbl)
        n1965 = Subtract(x=8.017352 ("y"), y=w2178) -> (x-y=w2185:dbl)
        n1966 = expression code="10**y"(w2191) -> (w2171:dbl)
        n1967 = expression code="10**y"(w2185) -> (w2184:dbl)
        n1968 = Multiply(x=w2169, y=w2171) -> (x*y=w2170:dbl)
        n1969 = Multiply(x=w2182, y=w2184) -> (x*y=w2183:dbl)
        n1970 = Divide(x=w2170, y=750.0) -> (x/y=w2186:dbl)
        n1971 = Divide(x=w2183, y=750.0) -> (x/y=w2187:dbl)
        n1972 = Add(x=w2186, y=w2187) -> (x+y=w2188:dbl)
        n1973 = Divide(x=w2188, y=2.0) -> (x/y=w2190:dbl)
        n1974 = local write "AVP"(w2190) -> ()
        n1975 = Subtract(x=1.4, y=w2190) -> (x-y=w2173:dbl)
        n1976 = local read "HCF"() -> (w2174:dbl)
      }
      frame Enabled {
      }
    }
    n1977 = case shown="True" "EDIT 3" {
      frame False {
      }
      frame True {
        n1978 = local write "EDIT 3"(FALSE ("EDIT 3")) -> ()
        n1979 = local write "Main Tab"(T2."About" ("Main Tab")) -> ()
      }
    }
    n1980 = case shown="True" w2145 {
      frame False {
      }
      frame True {
        n1981 = local write "Re-Initialise"(FALSE ("Re-Initialise")) -> ()
      }
    }
    n1982 = case shown="False" w2159 {
      frame False {
        n1983 = local read "stopT"() -> (w3164:bool)
        n1984 = case shown="True" w3164 {
          frame False {
          }
          frame True {
            w3165 = FALSE
            n1985 = local write "stopT"(w3165) -> ()
            n1986 = local write "st enable"(w3165) -> ()
          }
        }
      }
      frame True {
        "stopT" <- TRUE
      }
    }
    n1987 = case shown="False" w2157 {
      frame False {
      }
      frame True {
      }
    }
    n1988 = case shown="True" w2147 {
      frame False {
        n1989 = property on="Password 2" class="Str"("Visible"=FALSE) -> ()  [unwired: 2 in, 2 out]
        n1990 = local write "Password 2"("" ("Password")) -> ()
      }
      frame True {
        n1991 = property on="Password 2" class="Str"("Visible"=TRUE) -> ()  [unwired: 2 in, 2 out]
        n1992 = Equal?(x="Password 2", y="HFRR1234") -> (x = y?=w2280:bool)
        n1993 = case shown="True" w2280 {
          tunnel: "Password 2" -> [w2283 _]
          frame False {
            n1994 = String Length(string=w2283) -> (length=w2284:i32)
            n1995 = Greater Than 0?(x=w2284) -> (x > 0?=w2282:bool)
            n1996 = case shown="False" w2282 {
              frame False {
                n1997 = property on="Password 2" class="Str"("Caption.Text"="Password (Advance Setting)") -> ()  [unwired: 2 in, 2 out]
              }
              frame True {
                n1998 = property on="Password 2" class="Str"("Caption.Text"="Incorrect Password!") -> ()  [unwired: 2 in, 2 out]
              }
            }
          }
          frame True {
            n1999 = local write "EDIT 2"(FALSE ("EDIT 2")) -> ()
            n2000 = local write "Password 2"("" ("Password")) -> ()
            n2001 = local write "Main Tab"(T2."Advance" ("Main Tab")) -> ()
            n2002 = local write "Main Dashboard Buttons"(T1."Advance" ("Main Dashboard Buttons")) -> ()
          }
        }
      }
    }
    n2003 = case shown="True" "Prog Uno" {
      frame False {
      }
      frame True {
        n2004 = stacked-sequence {
          frame #0 {
            n2005 = Delete(path (use dialog)=path "C:/LAB-IQ-NXT/UNOCOMPILE.bat" ("working directory")) -> ()  [unwired: 4 in, 3 out]
          }
          frame #1 {
            n2006 = local read "Com Port 1"() -> (w2745:refnum<visa-resource-name>)
            n2007 = Concatenate Strings("cmd.exe /c \"mode " ("command line"), w2745, ":1200,n,8,1\"\n" ("command line")) -> (w2750:string)
            n2008 = Concatenate Strings(w2750, "CD\\\nCD WinDucom\navrdude -C avrdude.conf -v -patmega328p -carduino -P" ("command line"), w2745, " -b115200 -D -Uflash:w:UNO_V20.hex:i\n" ("command line"), "\r") -> (w2752:string)
            "STR" <- w2752
            n2009 = call <vilib>:"Write Characters To File.vi"("append to file? (new file:F)"=FALSE, "character string"=w2752, "file path (dialog if empty)"=path "C:/LAB-IQ/UNOCOMPILE.bat" ("working directory")) -> ()  [unwired: 2 in, 1 out]
          }
          frame #2 {
            n2010 = disable-structure shown="Disabled" {
              frame Disabled {
                w2756 = "cmd.exe  /c \"C:\\LAB-IQ-NXT\\UNOCOMPILE.bat\"" ("string")
                n2011 = local write "Prog Uno"(FALSE ("run minimized? (F)")) -> ()
                n2012 = call <vilib>:"System Exec.vi"("expected output size  (4096)"=u32 65535, "run minimized? (F)"=FALSE, "wait until completion? (T)"=TRUE ("run minimized? (F)"), "working directory"=path "C:/LAB-IQ-NXT", "standard input"=w2756, "command line"=w2756) -> ("error out"=w2755:errorcluster, "standard output"=→"String 42":string)  [unwired: 2 in, 2 out]
                "error out 3" <- w2755
                n2013 = flat-sequence {
                  tunnel: w2755 -> [_]
                  frame #0 {
                  }
                }
              }
              frame Enabled {
              }
            }
          }
        }
      }
    }
    n2014 = case shown="\"CEC F-096-A-06\"" "TEST STANDARD" {
      tunnel: [2.0 ("Set Temp") 0.0 ("Set Temp") 2.0 ("Set Temp") 0.0 ("Set Temp")] -> w2148
      frame "ASTM D6079", Default {
        w2702 = 50.0 ("Hz")
        w2703 = 53.0 ("Set Rh")
        w2705 = 1.0 ("Set Strk")
        w2704 = 60.0 ("Set Temp")
        # "astm hide"
        n2015 = local write "NORMAL LOAD"(200.0 ("NORMAL LOAD")) -> ()
        n2016 = local write "Set Strk"(w2705) -> ()
        n2017 = local write "Set Hz"(w2702) -> ()
        n2018 = local write "Set Temp"(w2704) -> ()
        n2019 = local write "Set Rh"(w2703) -> ()
        n2020 = local write "test time"(75.0 ("test time")) -> ()
        n2021 = local write "Set Stroke:"(w2705) -> ()
        n2022 = local write "Set Humidity:"(w2703) -> ()
        n2023 = local write "Set Frequency:"(w2702) -> ()
        n2024 = local write "Set Temperature:"(w2704) -> ()
        "Test Standard" <- "ASTM D6079" ("Test Standard 2")
      }
      frame "ISO 12156" {
        n2025 = local write "Set Strk"(1.0 ("Set Strk")) -> ()
        n2026 = local write "NORMAL LOAD"(200.0 ("NORMAL LOAD")) -> ()
        n2027 = local write "Set Temp"(60.0 ("Set Temp")) -> ()
        n2028 = local write "test time"(75.0 ("test time")) -> ()
        n2029 = local write "Set Hz"(50.0 ("Hz")) -> ()
        n2030 = local write "Set Rh"(53.0 ("Set Rh")) -> ()
      }
      frame "CEC F-096-A-06" {
        n2031 = local write "Set Strk"(1.0 ("Set Strk")) -> ()
        n2032 = local write "NORMAL LOAD"(200.0 ("NORMAL LOAD")) -> ()
        n2033 = local write "Set Temp"(60.0 ("Set Temp")) -> ()
        n2034 = local write "test time"(75.0 ("test time")) -> ()
        n2035 = local write "Set Hz"(50.0 ("Hz")) -> ()
        n2036 = local write "Set Rh"(53.0 ("Set Rh")) -> ()
      }
      frame "Custom" {
      }
    }
    n2037 = case shown="True" "Prog Due" {
      frame False {
      }
      frame True {
        n2038 = stacked-sequence {
          frame #0 {
            n2039 = Delete(path (use dialog)=path "C:/LAB-IQ/DUECOMPILE.bat" ("working directory")) -> ()  [unwired: 4 in, 3 out]
          }
          frame #1 {
            n2040 = disable-structure shown="Disabled" {
              frame Disabled {
                n2041 = local read "visa due"() -> (w2727:string)
                n2042 = Concatenate Strings("cmd.exe /c \"mode " ("command line"), w2727, ":1200,n,8,1\"\n" ("command line")) -> (w2732:string)
                n2043 = Concatenate Strings(w2732, "CD\\\nCD WinDucom\nTIMEOUT 1\n bossac.exe -i -d --port=" ("command line"), w2727, " -U false -e -w -v -b DUE.bin -R\n" ("command line"), "\r") -> (w2734:string)
                "concatenated string 2" <- w2734
                n2044 = call <vilib>:"Write Characters To File.vi"("append to file? (new file:F)"=FALSE, "character string"=w2734, "file path (dialog if empty)"=path "C:/LAB-IQ-NXT/DUECOMPILE.bat" ("working directory")) -> ()  [unwired: 2 in, 1 out]
              }
              frame Enabled {
              }
            }
          }
          frame #2 {
            # "C:\\LAB-IQ-NXT\\DUECOMPILE.bat"
            n2045 = disable-structure shown="Disabled" {
              frame Disabled {
                w2739 = "cmd.exe  /c \"C:\\LAB-IQ-NXT\\DUECOMPILE.bat\"" ("string")
                n2046 = call <vilib>:"System Exec.vi"("expected output size  (4096)"=u32 65535, "run minimized? (F)"=FALSE, "wait until completion? (T)"=TRUE ("run minimized? (F)"), "working directory"=path "C:/LAB-IQ-NXT", "standard input"=w2739, "command line"=w2739) -> ("error out"=w2738:errorcluster, "standard output"=→"String 44":string)  [unwired: 2 in, 2 out]
                "error out 4" <- w2738
                n2047 = flat-sequence {
                  tunnel: w2738 -> [_]
                  frame #0 {
                  }
                }
              }
              frame Enabled {
              }
            }
            n2048 = local write "Prog Due"(FALSE ("Prog Due")) -> ()
          }
        }
      }
    }
    n2049 = Or(x=w2144, y=w2142) -> (x .or. y?=w2143:bool)
    n2050 = case shown="\"About\"" w2141 {
      tunnel: [T23."Acquire" ("Main Tab") T23."Compare Files" ("Main Tab") T23."About" ("Main Tab")] -> w2155
      frame "Acquire", Default {
      }
      frame "Compare Files" {
      }
      frame "About" {
      }
    }
    n2051 = Or(x=w2149, y="OPEN") -> (x .or. y?=w2150:bool)
    n2052 = case shown="True" w2150 {
      tunnel: w2149 -> [_ w2291]
      frame False {
      }
      frame True {
        n2053 = stacked-sequence {
          tunnel: w2291 -> [_ w2358 _ _]
          frame #0 {
            w2307 = "  " ("String 6")
            n2054 = local write "OPEN"(FALSE ("open")) -> ()
            n2055 = local read "string1 2"() -> (w2295:string)
            n2056 = local read "string1 3"() -> (w2294:string)
            n2057 = local read "string1 4"() -> (w2293:string)
            n2058 = property on="OPEN" class="Bool (strict)"("Visible"=FALSE) -> ()  [unwired: 2 in, 2 out]
            n2059 = local write "String 6"(w2307) -> ()
            n2060 = local write "String 7"(w2307) -> ()
            n2061 = local write "String 8"(w2307) -> ()
            n2062 = local write "String 12"(w2307) -> ()
            n2063 = local read "OK Button 16"() -> (w2292:bool)
            n2064 = String To Path(string=w2295) -> (path=w2303:path)
            n2065 = String To Path(string=w2294) -> (path=w2302:path)
            n2066 = String To Path(string=w2293) -> (path=w2301:path)
            n2067 = case shown="True" w2292 {
              tunnel: [w2308 w2309] -> w2296
              frame False {
                n2068 = local read "string1"() -> (w2308:string)
              }
              frame True {
                n2069 = local read "String Indicator 4"() -> (w2309:string)
              }
            }
            n2070 = Open/Create/Replace File "Open File"(file path (use dialog)=w2303) -> (refnum out=w2299:refnum<file>)  [unwired: 5 in, 2 out]
            n2071 = Open/Create/Replace File "Open File"(file path (use dialog)=w2302) -> (refnum out=w2298:refnum<file>)  [unwired: 5 in, 2 out]
            n2072 = Open/Create/Replace File "Open File"(file path (use dialog)=w2301) -> (refnum out=w2297:refnum<file>)  [unwired: 5 in, 2 out]
            n2073 = while {
              tunnel: w2299 -> [w2321]
              i -> [w2317]
              stop <- w2316 continue-if-true
              (unwired) TRUE ("line mode (F)")
              n2074 = Read from Text File "Read File"(file (use dialog)=w2321) -> (text=w2318:string)  [unwired: 3 in, 3 out]
              n2075 = local write "Numeric 11"(w2317) -> ()
              n2076 = String Length(string=w2318) -> (length=w2320:i32)
              n2077 = Greater?(x=w2320, y=1) -> (0:w2316:bool)
            }
            n2078 = while {
              tunnel: w2298 -> [w2327]
              i -> [w2323]
              stop <- w2322 continue-if-true
              (unwired) TRUE ("line mode (F)")
              n2079 = Read from Text File "Read File"(file (use dialog)=w2327) -> (text=w2324:string)  [unwired: 3 in, 3 out]
              n2080 = local write "Numeric 12"(w2323) -> ()
              n2081 = String Length(string=w2324) -> (length=w2326:i32)
              n2082 = Greater?(x=w2326, y=1) -> (0:w2322:bool)
            }
            n2083 = while {
              tunnel: w2297 -> [w2333]
              i -> [w2329]
              stop <- w2328 continue-if-true
              (unwired) TRUE ("line mode (F)")
              n2084 = Read from Text File "Read File"(file (use dialog)=w2333) -> (text=w2330:string)  [unwired: 3 in, 3 out]
              n2085 = local write "Numeric 13"(w2329) -> ()
              n2086 = String Length(string=w2330) -> (length=w2332:i32)
              n2087 = Greater?(x=w2332, y=1) -> (0:w2328:bool)
            }
            n2088 = String To Path(string=w2296) -> (path=w2304:path)
            n2089 = Open/Create/Replace File "Open File"(file path (use dialog)=w2304) -> (refnum out=w2300:refnum<file>)  [unwired: 5 in, 2 out]
            n2090 = while {
              tunnel: w2300 -> [w2315]
              i -> [w2311]
              stop <- w2310 continue-if-true
              (unwired) TRUE ("line mode (F)")
              n2091 = Read from Text File "Read File"(file (use dialog)=w2315) -> (text=w2312:string)  [unwired: 3 in, 3 out]
              n2092 = local write "Numeric 8"(w2311) -> ()
              n2093 = String Length(string=w2312) -> (length=w2314:i32)
              n2094 = Greater?(x=w2314, y=1) -> (0:w2310:bool)
            }
          }
          frame #1 {
            w2485 = FALSE ("ACTUAL   MERGE")
            # "Sample Temp"
            # "ECR"
            # "COF"
            # "Time\nCOF\nFF\nTemp"
            n2095 = case shown="True" w2358 {
              tunnel: [w2505 w2506] -> w2359
              frame False {
                n2096 = local read "string1"() -> (w2505:string)
              }
              frame True {
                n2097 = local read "String Indicator 4"() -> (w2506:string)
              }
            }
            n2098 = local read "string1 3"() -> (w2403:string)
            n2099 = String To Path(string=w2359) -> (path=w2490:path)
            n2100 = String To Path(string=w2403) -> (path=w2501:path)
            n2101 = local read "Numeric 12"() -> (w2487:i32)
            n2102 = local read "Numeric 8"() -> (w2489:i32)
            n2103 = local read "string1 2"() -> (w2404:string)
            n2104 = local read "string1 4"() -> (w2402:string)
            n2105 = Open/Create/Replace File "Open File"(file path (use dialog)=w2490) -> (refnum out=w2504:refnum<file>, error out=w2503:errorcluster)  [unwired: 5 in, 1 out]
            n2106 = Open/Create/Replace File "Open File"(file path (use dialog)=w2501) -> (refnum out=w2497:refnum<file>, error out=w2498:errorcluster)  [unwired: 5 in, 1 out]
            n2107 = for {
              N: w2489 -> [_]
              tunnel: w2504 -> [w2652]
              tunnel: w2503 -> [w2651]
              tunnel: [w2641] -> w2416 mode=indexing
              tunnel: [w2639] -> w2473 mode=indexing
              tunnel: [w2640] -> w2468 mode=indexing
              tunnel: w2485 -> [_]
              tunnel: [w2633] -> w2470 mode=indexing
              tunnel: [w2629] -> w2439 mode=indexing
              tunnel: [w2625] -> w2414 mode=indexing
              tunnel: [w2621] -> w2395 mode=indexing
              tunnel: [w2616] -> w2355 mode=indexing
              (unwired) TRUE ("line mode (F)")
              # "freq"
              # "Stroke"
              # "Time"
              # "CoF"
              # "Humidity"
              # "Temp"
              # "Air Temp"
              # "ECR"
              n2108 = Read from Text File "Read File"(file (use dialog)=w2652, error in=w2651) -> (text=w2617:string)  [unwired: 2 in, 3 out]
              n2109 = local write "String 6"(w2617) -> ()
              n2110 = String Subset(string=w2617, offset (0)=0, length (rest)=14 ("length (rest)")) -> (substring=w2645:string)
              n2111 = String Subset(string=w2617, offset (0)=35, length (rest)=9 ("length (rest)")) -> (substring=w2642:string)
              n2112 = String Subset(string=w2617, offset (0)=15, length (rest)=9 ("length (rest)")) -> (substring=w2648:string)
              n2113 = Fract/Exp String To Number(string=w2645) -> (number=w2641:dbl)  [unwired: 3 in, 1 out]
              n2114 = Fract/Exp String To Number(string=w2642) -> (number=w2640:dbl)  [unwired: 3 in, 1 out]
              n2115 = Fract/Exp String To Number(string=w2648) -> (number=w2639:dbl)  [unwired: 3 in, 1 out]
              n2116 = String Subset(string=w2617, offset (0)=85, length (rest)=9 ("length (rest)")) -> (substring=w2618:string)
              n2117 = String Subset(string=w2617, offset (0)=25, length (rest)=9 ("length (rest)")) -> (substring=w2624:string)
              n2118 = String Subset(string=w2617, offset (0)=55, length (rest)=9 ("length (rest)")) -> (substring=w2626:string)
              n2119 = String Subset(string=w2617, offset (0)=45, length (rest)=9 ("length (rest)")) -> (substring=w2632:string)
